vi "Secret Suprise.vi"() -> ()   [LabVIEW 2016]
uses:
  <vilib>/Rock Robotics/WPI/Utilities/WPI_GetSetVariantRefNum.vi
  SUPPORT/Secret.vi
panel:
  out "Secret":bool
  out "Suprise":bool
  out "Number":dbl
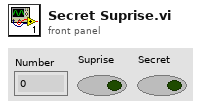
[diagram p1: front panel]
types:
  T1 = typedef "WPI_JoystickDevRef.ctl" = cluster{"Device":T2}
  T2 = typedef "WPI_JoystickDeviceEnum.ctl" = enum16{"USB 0", "USB 1", "USB 2", "USB 3", "USB 4", "USB 5"}
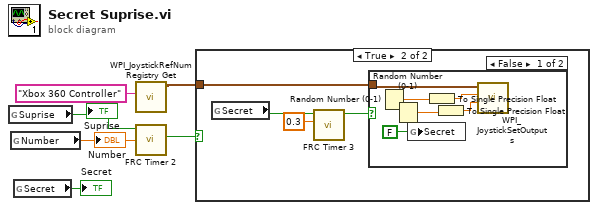
[diagram p0: block diagram]
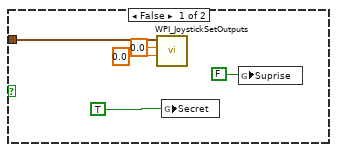
[diagram p2: hidden frame]
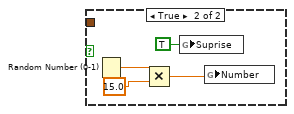
[diagram p3: hidden frame]
diagram:
  n1 = global read "Secret.vi" "Suprise"() -> (w2:bool)
  "Suprise" <- w2
  n2 = global read "Secret.vi" "Number"() -> (w3:dbl)
  "Number" <- w3
  n3 = global read "Secret.vi" "Secret"() -> (→"Secret":bool)
  n4 = call <vilib>:"WPI_JoystickRefNum Registry Get.vi"("refnum name"="Xbox 360 Controller") -> ("JoystickDevRef"=w5:T1)  [unwired: 9 in, 1 out]
  n5 = call "FRC Timer 2.vi"("Time Target (s)"=w3, "Boolean"=w2) -> ("Has Time Elapsed"=w4:bool)  [unwired: 7 in, 2 out]
  n6 = case shown="True" w4 {
    tunnel: w5 -> [w10 w15]
    frame False {
      n7 = call <vilib>:"WPI_JoystickSetOutputs.vi"("Right Rumble"=sgl 0.0, "Left Rumble"=sgl 0.0, "JoystickDevRef"=w10) -> ()  [unwired: 7 in, 2 out]
      n8 = global write "Secret.vi" "Secret"(TRUE) -> ()
      n9 = global write "Secret.vi" "Suprise"(FALSE) -> ()
    }
    frame True {
      n10 = global read "Secret.vi" "Secret"() -> (w13:bool)
      n11 = call "FRC Timer 3.vi"("Time Target (s)"=0.3, "Boolean"=w13) -> ("Has Time Elapsed"=w14:bool)  [unwired: 7 in, 2 out]
      n12 = case shown="False" w14 {
        tunnel: w15 -> [w21 _]
        frame False {
          n13 = Random Number (0-1)() -> (number: 0 to 1=w18:dbl)
          n14 = Random Number (0-1)() -> (number: 0 to 1=w17:dbl)
          n15 = global write "Secret.vi" "Secret"(FALSE) -> ()
          n16 = To Single Precision Float(number=w18) -> (single precision float=w19:sgl)
          n17 = To Single Precision Float(number=w17) -> (single precision float=w16:sgl)
          n18 = call <vilib>:"WPI_JoystickSetOutputs.vi"("Right Rumble"=w16, "Left Rumble"=w19, "JoystickDevRef"=w21) -> ()  [unwired: 7 in, 2 out]
        }
        frame True {
          n19 = Random Number (0-1)() -> (number: 0 to 1=w24:dbl)
          n20 = Multiply(x=w24, y=15.0) -> (x*y=w22:dbl)
          n21 = global write "Secret.vi" "Suprise"(TRUE) -> ()
          n22 = global write "Secret.vi" "Number"(w22) -> ()
        }
      }
    }
  }
